vi "To SRational.vi"(3 "Number":dbl) -> (0 "Denominator":i32, 1 "Numerator":i32)   [LabVIEW 2020, in "LV Tiff.lvlib"]
uses:
  LV Tiff.lvlib
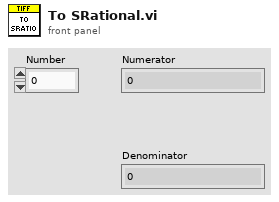
[diagram p1: front panel]
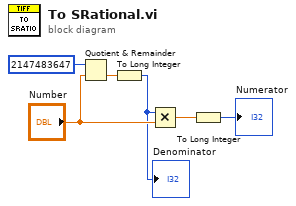
[diagram p0: block diagram]
diagram:
  n1 = Quotient & Remainder(x=2147483647, y="Number") -> (floor(x/y)=w3:dbl)  [unwired: 1 out]
  n2 = To Long Integer(number=w3) -> (32bit integer=w2:i32)
  "Denominator" <- w2
  n3 = Multiply(x=w2, y="Number") -> (x*y=w4:dbl)
  n4 = To Long Integer(number=w4) -> (32bit integer=→"Numerator":i32)
